vi "Disconnect.vi"(8 "error in (no error)":errorcluster, 11 "Network Actor in":refnum<class "Client Proxy LNA.lvclass">) -> (0 "error out":errorcluster, 3 "Network Actor out":refnum<class "Client Proxy LNA.lvclass">)   [LabVIEW 2017, in "Client Proxy LNA.lvlib" / "Client Proxy LNA.lvclass"]
doc: "If the local writer stream is connected, flushes the message queue. Destroys the local writer stream."
uses:
  Client Proxy LNA.lvclass
  C:/Program Files (x86)/National Instruments/LabVIEW 2017/vi.lib/ActorFramework/Actor/Actor.lvclass
  <vilib>/ActorFramework/Actor/Actor.lvclass/Actor.ctl
  <vilib>/ActorFramework/Message Enqueuer/Message Enqueuer.lvclass/Message Enqueuer.ctl
  <vilib>/ActorFramework/Message Enqueuer/Enqueue.vi
  <vilib>/ActorFramework/Message Enqueuer/Init from Existing Queue.vi
  <vilib>/ActorFramework/Stop Msg/Stop Msg.lvclass
  C:/Program Files (x86)/National Instruments/LabVIEW 2017/vi.lib/ActorFramework/Message/Message.lvclass
  <vilib>/ActorFramework/Message Priority Queue/Priority Enqueue.vi
  <vilib>/NI/Actors/Linked Network Actor/Linked Network Actor/Linked Network Actor.lvclass
  <vilib>/ActorFramework/Message Enqueuer/Message Enqueuer.lvclass
  <vilib>/ActorFramework/Actor/Actor.lvclass
  MAL-Framework/user.lib/Common Components/Controller/Messages/Log Status/Log Status.lvclass
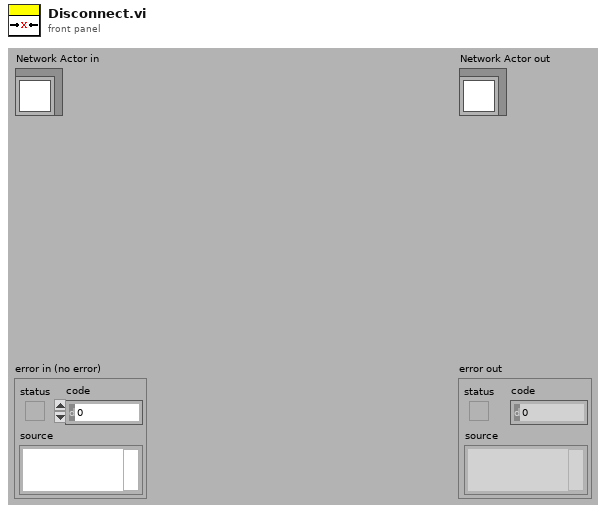
[diagram p1: front panel]
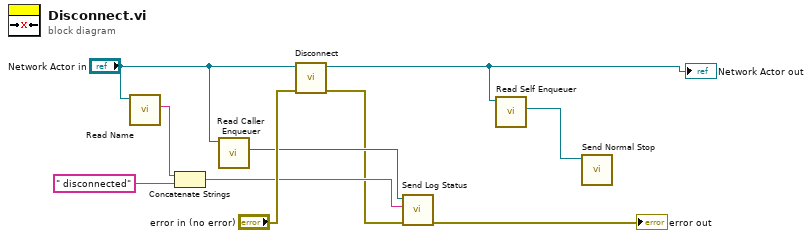
[diagram p0: block diagram]
diagram:
  n1 = call-dynamic "Read Name.vi"("Network Actor in"="Network Actor in") -> ("Name"=w6:string)  [unwired: 10 in]
  n2 = Concatenate Strings(w6, " disconnected" ("string")) -> (w8:string)
  n3 = call <vilib>:"Read Caller Enqueuer.vi"("Actor"="Network Actor in") -> ("Caller Enqueuer"=w9:refnum<class "Message Enqueuer.lvclass">)  [unwired: 10 in]
  n4 = call-parent "Disconnect.vi"("error in (no error)"="error in (no error)", "Network Actor in"="Network Actor in") -> ("error out"=w4:errorcluster, "Network Actor out"=w2:refnum<class "Client Proxy LNA.lvclass">)  [unwired: 8 in]
  "Network Actor out" <- w2
  n5 = call "Send Log Status.vi"("error in (no error)"=w4, "String"=w8, "Message Enqueuer in"=w9) -> ("error out"=→"error out":errorcluster)  [unwired: 7 in, 1 out]
  n6 = call <vilib>:"Read Self Enqueuer.vi"("Actor"=w2) -> ("Self Enqueuer"=w3:refnum<class "Message Enqueuer.lvclass">)  [unwired: 10 in]
  n7 = call <vilib>:"Send Normal Stop.vi"("Message Enqueuer"=w3) -> ()  [unwired: 10 in, 1 out]
